vi "VISJS Viewer.vi"(4 "Extra Scripts":string, 5 "FileDependency out":map{path, T1}(c390), 6 "Options":string, 7 "OpenWebBrowser(False)":bool, 8 "error in":errorcluster, 9 "Embedd VISJS Librarya in HTMl File(False)":bool, 10 "HTMLFilePath":path, 11 "LibraryDependency":map{path, T3}(c390)) -> (0 "error out":errorcluster, 3 "HTMLFileContent":string)   [LabVIEW 2020, in "VISJS Viewer.lvlib"] (continued)
this.physicsBody,g),this.gravitySolver=new WR(this.body,this.physicsBody,g)):\"hierarchicalRepulsion\"===this.options.solver?(g=this.options.hierarchicalRepulsion,this.nodesSolver=new LR(this.body,this.physicsBody,g),this.edgesSolver=new YR(this.body,this.physicsBody,g),this.gravitySolver=new WR(this.body,this.physicsBody,g)):(g=this.options.barnesHut,this.nodesSolver=new GR(this.body,this.physicsBody,g),this.edgesSolver=new VR(this.body,this.physicsBody,g),this.gravitySolver=new WR(this.body,this.physicsBody,g)),this.modelOptions=g}},{key:\"initPhysics\",value:function(){!0===this.physicsEnabled&&!0===this.options.enabled?!0===this.options.stabilization.enabled?this.stabilize():(this.stabilized=!1,this.ready=!0,this.body.emitter.emit(\"fit\",{},this.layoutFailed),this.startSimulation()):(this.ready=!0,this.body.emitter.emit(\"fit\"))}},{key:\"startSimulation\",value:function(){var g;!0===this.physicsEnabled&&!0===this.options.enabled?(this.stabilized=!1,this.adaptiveTimestep=!1,this.body.emitter.emit(\"_resizeNodes\"),void 0===this.viewFunction&&(this.viewFunction=je(g=this.simulationStep).call(g,this),this.body.emitter.on(\"initRedraw\",this.viewFunction),this.body.emitter.emit(\"_startRendering\"))):this.body.emitter.emit(\"_redraw\")}},{key:\"stopSimulation\",value:function(){var g=!(arguments.length>0&&void 0!==arguments[0])||arguments[0];this.stabilized=!0,!0===g&&this._emitStabilized(),void 0!==this.viewFunction&&(this.body.emitter.off(\"initRedraw\",this.viewFunction),this.viewFunction=void 0,!0===g&&this.body.emitter.emit(\"_stopRendering\"))}},{key:\"simulationStep\",value:function(){var g=Qh();this.physicsTick(),(Qh()-g<.4*this.simulationInterval||!0===this.runDoubleSpeed)&&!1===this.stabilized&&(this.physicsTick(),this.runDoubleSpeed=!0),!0===this.stabilized&&this.stopSimulation()}},{key:\"_emitStabilized\",value:function(){var g=this,t=arguments.length>0&&void 0!==arguments[0]?arguments[0]:this.stabilizationIterations;(this.stabilizationIterations>1||!0===this.startedStabilization)&&wu((function(){g.body.emitter.emit(\"stabilized\",{iterations:t}),g.startedStabilization=!1,g.stabilizationIterations=0}),0)}},{key:\"physicsStep\",value:function(){this.gravitySolver.solve(),this.nodesSolver.solve(),this.edgesSolver.solve(),this.moveNodes()}},{key:\"adjustTimeStep\",value:function(){!0===this._evaluateStepQuality()?this.timestep=1.2*this.timestep:this.timestep/1.2<this.options.timestep?this.timestep=this.options.timestep:(this.adaptiveCounter=-1,this.timestep=Math.max(this.options.timestep,this.timestep/1.2))}},{key:\"physicsTick\",value:function(){if(this._startStabilizing(),!0!==this.stabilized){if(!0===this.adaptiveTimestep&&!0===this.adaptiveTimestepEnabled)this.adaptiveCounter%this.adaptiveInterval==0?(this.timestep=2*this.timestep,this.physicsStep(),this.revert(),this.timestep=.5*this.timestep,this.physicsStep(),this.physicsStep(),this.adjustTimeStep()):this.physicsStep(),this.adaptiveCounter+=1;else this.timestep=this.options.timestep,this.physicsStep();!0===this.stabilized&&this.revert(),this.stabilizationIterations++}}},{key:\"updatePhysicsData\",value:function(){this.physicsBody.forces={},this.physicsBody.physicsNodeIndices=[],this.physicsBody.physicsEdgeIndices=[];var g=this.body.nodes,t=this.body.edges;for(var A in g)Object.prototype.hasOwnProperty.call(g,A)&&!0===g[A].options.physics&&this.physicsBody.physicsNodeIndices.push(g[A].id);for(var e in t)Object.prototype.hasOwnProperty.call(t,e)&&!0===t[e].options.physics&&this.physicsBody.physicsEdgeIndices.push(t[e].id);for(var C=0;C<this.physicsBody.physicsNodeIndices.length;C++){var I=this.physicsBody.physicsNodeIndices[C];this.physicsBody.forces[I]={x:0,y:0},void 0===this.physicsBody.velocities[I]&&(this.physicsBody.velocities[I]={x:0,y:0})}for(var i in this.physicsBody.velocities)void 0===g[i]&&delete this.physicsBody.velocities[i]}},{key:\"revert\",value:function(){var g=Lh(this.previousStates),t=this.body.nodes,A=this.physicsBody.velocities;this.referenceState={};for(var e=0;e<g.length;e++){var C=g[e];void 0!==t[C]?!0===t[C].options.physics&&(this.referenceState[C]={positions:{x:t[C].x,y:t[C].y}},A[C].x=this.previousStates[C].vx,A[C].y=this.previousStates[C].vy,t[C].x=this.previousStates[C].x,t[C].y=this.previousStates[C].y):delete this.previousStates[C]}}},{key:\"_evaluateStepQuality\",value:function(){var g,t,A=this.body.nodes,e=this.referenceState;for(var C in this.referenceState)if(Object.prototype.hasOwnProperty.call(this.referenceState,C)&&void 0!==A[C]&&(g=A[C].x-e[C].positions.x,t=A[C].y-e[C].positions.y,Math.sqrt(Math.pow(g,2)+Math.pow(t,2))>.3))return!1;return!0}},{key:\"moveNodes\",value:function(){for(var g=this.physicsBody.physicsNodeIndices,t=0,A=0,e=0;e<g.length;e++){var C=g[e],I=this._performStep(C);t=Math.max(t,I),A+=I}this.adaptiveTimestepEnabled=A/g.length<5,this.stabilized=t<this.options.minVelocity}},{key:\"calculateComponentVelocity\",value:function(g,t,A){g+=(t-this.modelOptions.damping*g)/A*this.timestep;var e=this.options.maxVelocity||1e9;return Math.abs(g)>e&&(g=g>0?e:-e),g}},{key:\"_performStep\",value:function(g){var t=this.body.nodes[g],A=this.physicsBody.forces[g];this.options.wind&&(A.x+=this.options.wind.x,A.y+=this.options.wind.y);var e=this.physicsBody.velocities[g];return this.previousStates[g]={x:t.x,y:t.y,vx:e.x,vy:e.y},!1===t.options.fixed.x?(e.x=this.calculateComponentVelocity(e.x,A.x,t.options.mass),t.x+=e.x*this.timestep):(A.x=0,e.x=0),!1===t.options.fixed.y?(e.y=this.calculateComponentVelocity(e.y,A.y,t.options.mass),t.y+=e.y*this.timestep):(A.y=0,e.y=0),Math.sqrt(Math.pow(e.x,2)+Math.pow(e.y,2))}},{key:\"_freezeNodes\",value:function(){var g=this.body.nodes;for(var t in g)if(Object.prototype.hasOwnProperty.call(g,t)&&g[t].x&&g[t].y){var A=g[t].options.fixed;this.freezeCache[t]={x:A.x,y:A.y},A.x=!0,A.y=!0}}},{key:\"_restoreFrozenNodes\",value:function(){var g=this.body.nodes;for(var t in g)Object.prototype.hasOwnProperty.call(g,t)&&void 0!==this.freezeCache[t]&&(g[t].options.fixed.x=this.freezeCache[t].x,g[t].options.fixed.y=this.freezeCache[t].y);this.freezeCache={}}},{key:\"stabilize\",value:function(){var g=this,t=arguments.length>0&&void 0!==arguments[0]?arguments[0]:this.options.stabilization.iterations;\"number\"!=typeof t&&(t=this.options.stabilization.iterations,console.error(\"The stabilize method needs a numeric amount of iterations. Switching to default: \",t)),0!==this.physicsBody.physicsNodeIndices.length?(this.adaptiveTimestep=this.options.adaptiveTimestep,this.body.emitter.emit(\"_resizeNodes\"),this.stopSimulation(),this.stabilized=!1,this.body.emitter.emit(\"_blockRedraw\"),this.targetIterations=t,!0===this.options.stabilization.onlyDynamicEdges&&this._freezeNodes(),this.stabilizationIterations=0,wu((function(){return g._stabilizationBatch()}),0)):this.ready=!0}},{key:\"_startStabilizing\",value:function(){return!0!==this.startedStabilization&&(this.body.emitter.emit(\"startStabilizing\"),this.startedStabilization=!0,!0)}},{key:\"_stabilizationBatch\",value:function(){var g=this,t=function(){return!1===g.stabilized&&g.stabilizationIterations<g.targetIterations},A=function(){g.body.emitter.emit(\"stabilizationProgress\",{iterations:g.stabilizationIterations,total:g.targetIterations})};this._startStabilizing()&&A();for(var e,C=0;t()&&C<this.options.stabilization.updateInterval;)this.physicsTick(),C++;(A(),t())?wu(je(e=this._stabilizationBatch).call(e,this),0):this._finalizeStabilization()}},{key:\"_finalizeStabilization\",value:function(){this.body.emitter.emit(\"_allowRedraw\"),!0===this.options.stabilization.fit&&this.body.emitter.emit(\"fit\"),!0===this.options.stabilization.onlyDynamicEdges&&this._restoreFrozenNodes(),this.body.emitter.emit(\"stabilizationIterationsDone\"),this.body.emitter.emit(\"_requestRedraw\"),!0===this.stabilized?this._emitStabilized():this.startSimulation(),this.ready=!0}},{key:\"_drawForces\",value:function(g){for(var t=0;t<this.physicsBody.physicsNodeIndices.length;t++){var A=this.physicsBody.physicsNodeIndices[t],e=this.body.nodes[A],C=this.physicsBody.forces[A],I=Math.sqrt(Math.pow(C.x,2)+Math.pow(C.x,2)),i=Math.min(Math.max(5,I),15),o=3*i,n=nv((180-180*Math.min(1,Math.max(0,.03*I)))/360,1,1),r={x:e.x+20*C.x,y:e.y+20*C.y};g.lineWidth=i,g.strokeStyle=n,g.beginPath(),g.moveTo(e.x,e.y),g.lineTo(r.x,r.y),g.stroke();var s=Math.atan2(C.y,C.x);g.fillStyle=n,vR.draw(g,{type:\"arrow\",point:r,angle:s,length:o}),Bu(g).call(g)}}}]),g}(),XR=function(){function g(){cn(this,g)}return kd(g,null,[{key:\"getRange\",value:function(g){var t,A=arguments.length>1&&void 0!==arguments[1]?arguments[1]:[],e=1e9,C=-1e9,I=1e9,i=-1e9;if(A.length>0)for(var o=0;o<A.length;o++)I>(t=g[A[o]]).shape.boundingBox.left&&(I=t.shape.boundingBox.left),i<t.shape.boundingBox.right&&(i=t.shape.boundingBox.right),e>t.shape.boundingBox.top&&(e=t.shape.boundingBox.top),C<t.shape.boundingBox.bottom&&(C=t.shape.boundingBox.bottom);return 1e9===I&&-1e9===i&&1e9===e&&-1e9===C&&(e=0,C=0,I=0,i=0),{minX:I,maxX:i,minY:e,maxY:C}}},{key:\"getRangeCore\",value:function(g){var t,A=arguments.length>1&&void 0!==arguments[1]?arguments[1]:[],e=1e9,C=-1e9,I=1e9,i=-1e9;if(A.length>0)for(var o=0;o<A.length;o++)I>(t=g[A[o]]).x&&(I=t.x),i<t.x&&(i=t.x),e>t.y&&(e=t.y),C<t.y&&(C=t.y);return 1e9===I&&-1e9===i&&1e9===e&&-1e9===C&&(e=0,C=0,I=0,i=0),{minX:I,maxX:i,minY:e,maxY:C}}},{key:\"findCenter\",value:function(g){return{x:.5*(g.maxX+g.minX),y:.5*(g.maxY+g.minY)}}},{key:\"cloneOptions\",value:function(g,t){var A={};return void 0===t||\"node\"===t?(qf(A,g.options,!0),A.x=g.x,A.y=g.y,A.amountOfConnections=g.edges.length):qf(A,g.options,!0),A}}]),g}();function JR(g){var t=function(){if(\"undefined\"==typeof Reflect||!MT)return!1;if(MT.sham)return!1;if(\"function\"==typeof Proxy)return!0;try{return Boolean.prototype.valueOf.call(MT(Boolean,[],(function(){}))),!0}catch(g){return!1}}();return function(){var A,e=nb(g);if(t){var C=nb(this).constructor;A=MT(e,arguments,C)}else A=e.apply(this,arguments);return Ib(this,A)}}var qR=function(g){Cb(A,g);var t=JR(A);function A(g,e,C,I,i,o){var n;return cn(this,A),(n=t.call(this,g,e,C,I,i,o)).isCluster=!0,n.containedNodes={},n.containedEdges={},n}return kd(A,[{key:\"_openChildCluster\",value:function(g){var t=this,A=this.body.nodes[g];if(void 0===this.containedNodes[g])throw new Error(\"node with id: \"+g+\" not in current cluster\");if(!A.isCluster)throw new Error(\"node with id: \"+g+\" is not a cluster\");delete this.containedNodes[g],tv(A.edges,(function(g){delete t.containedEdges[g.id]})),tv(A.containedNodes,(function(g,A){t.containedNodes[A]=g})),A.containedNodes={},tv(A.containedEdges,(function(g,A){t.containedEdges[A]=g})),A.containedEdges={},tv(A.edges,(function(g){tv(t.edges,(function(A){var e,C,I=Xc(e=A.clusteringEdgeReplacingIds).call(e,g.id);-1!==I&&(tv(g.clusteringEdgeReplacingIds,(function(g){A.clusteringEdgeReplacingIds.push(g),t.body.edges[g].edgeReplacedById=A.id})),Zl(C=A.clusteringEdgeReplacingIds).call(C,I,1))}))})),A.edges=[]}}]),A}(jN),$R=function(){function g(t){var A=this;cn(this,g),this.body=t,this.clusteredNodes={},this.clusteredEdges={},this.options={},this.defaultOptions={},fe(this.options,this.defaultOptions),this.body.emitter.on(\"_resetData\",(function(){A.clusteredNodes={},A.clusteredEdges={}}))}return kd(g,[{key:\"clusterByHubsize\",value:function(g,t){void 0===g?g=this._getHubSize():\"object\"===yd(g)&&(t=this._checkOptions(g),g=this._getHubSize());for(var A=[],e=0;e<this.body.nodeIndices.length;e++){var C=this.body.nodes[this.body.nodeIndices[e]];C.edges.length>=g&&A.push(C.id)}for(var I=0;I<A.length;I++)this.clusterByConnection(A[I],t,!0);this.body.emitter.emit(\"_dataChanged\")}},{key:\"cluster\",value:function(){var g=this,t=arguments.length>0&&void 0!==arguments[0]?arguments[0]:{},A=!(arguments.length>1&&void 0!==arguments[1])||arguments[1];if(void 0===t.joinCondition)throw new Error(\"Cannot call clusterByNodeData without a joinCondition function in the options.\");t=this._checkOptions(t);var e={},C={};tv(this.body.nodes,(function(A,I){A.options&&!0===t.joinCondition(A.options)&&(e[I]=A,tv(A.edges,(function(t){void 0===g.clusteredEdges[t.id]&&(C[t.id]=t)})))})),this._cluster(e,C,t,A)}},{key:\"clusterByEdgeCount\",value:function(g,t){var A=this,e=!(arguments.length>2&&void 0!==arguments[2])||arguments[2];t=this._checkOptions(t);for(var C,I,i,o=[],n={},r=function(){var e={},r={},a=A.body.nodeIndices[s],d=A.body.nodes[a];if(void 0===n[a]){i=0,I=[];for(var h=0;h<d.edges.length;h++)C=d.edges[h],void 0===A.clusteredEdges[C.id]&&(C.toId!==C.fromId&&i++,I.push(C));if(i===g){for(var l=function(g){if(void 0===t.joinCondition||null===t.joinCondition)return!0;var A=XR.cloneOptions(g);return t.joinCondition(A)},c=!0,u=0;u<I.length;u++){C=I[u];var p=A._getConnectedId(C,a);if(!l(d)){c=!1;break}r[C.id]=C,e[a]=d,e[p]=A.body.nodes[p],n[a]=!0}if(Lh(e).length>0&&Lh(r).length>0&&!0===c){var f=function(){for(var g=0;g<o.length;++g)for(var t in e)if(void 0!==o[g].nodes[t])return o[g]}();if(void 0!==f){for(var v in e)void 0===f.nodes[v]&&(f.nodes[v]=e[v]);for(var y in r)void 0===f.edges[y]&&(f.edges[y]=r[y])}else o.push({nodes:e,edges:r})}}}},s=0;s<this.body.nodeIndices.length;s++)r();for(var a=0;a<o.length;a++)this._cluster(o[a].nodes,o[a].edges,t,!1);!0===e&&this.body.emitter.emit(\"_dataChanged\")}},{key:\"clusterOutliers\",value:function(g){var t=!(arguments.length>1&&void 0!==arguments[1])||arguments[1];this.clusterByEdgeCount(1,g,t)}},{key:\"clusterBridges\",value:function(g){var t=!(arguments.length>1&&void 0!==arguments[1])||arguments[1];this.clusterByEdgeCount(2,g,t)}},{key:\"clusterByConnection\",value:function(g,t){var A,e=!(arguments.length>2&&void 0!==arguments[2])||arguments[2];if(void 0===g)throw new Error(\"No nodeId supplied to clusterByConnection!\");if(void 0===this.body.nodes[g])throw new Error(\"The nodeId given to clusterByConnection does not exist!\");var C=this.body.nodes[g];void 0===(t=this._checkOptions(t,C)).clusterNodeProperties.x&&(t.clusterNodeProperties.x=C.x),void 0===t.clusterNodeProperties.y&&(t.clusterNodeProperties.y=C.y),void 0===t.clusterNodeProperties.fixed&&(t.clusterNodeProperties.fixed={},t.clusterNodeProperties.fixed.x=C.options.fixed.x,t.clusterNodeProperties.fixed.y=C.options.fixed.y);var I={},i={},o=C.id,n=XR.cloneOptions(C);I[o]=C;for(var r=0;r<C.edges.length;r++){var s=C.edges[r];if(void 0===this.clusteredEdges[s.id]){var a=this._getConnectedId(s,o);if(void 0===this.clusteredNodes[a])if(a!==o)if(void 0===t.joinCondition)i[s.id]=s,I[a]=this.body.nodes[a];else{var d=XR.cloneOptions(this.body.nodes[a]);!0===t.joinCondition(n,d)&&(i[s.id]=s,I[a]=this.body.nodes[a])}else i[s.id]=s}}var h=Fh(A=Lh(I)).call(A,(function(g){return I[g].id}));for(var l in I)if(Object.prototype.hasOwnProperty.call(I,l))for(var c=I[l],u=0;u<c.edges.length;u++){var p=c.edges[u];Xc(h).call(h,this._getConnectedId(p,c.id))>-1&&(i[p.id]=p)}this._cluster(I,i,t,e)}},{key:\"_createClusterEdges\",value:function(g,t,A,e){for(var C,I,i,o,n,r,s=Lh(g),a=[],d=0;d<s.length;d++){i=g[I=s[d]];for(var h=0;h<i.edges.length;h++)C=i.edges[h],void 0===this.clusteredEdges[C.id]&&(C.toId==C.fromId?t[C.id]=C:C.toId==I?(o=A.id,r=n=C.fromId):(o=C.toId,n=A.id,r=o),void 0===g[r]&&a.push({edge:C,fromId:n,toId:o}))}for(var l=[],c=function(g){for(var t=0;t<l.length;t++){var A=l[t],e=g.fromId===A.fromId&&g.toId===A.toId,C=g.fromId===A.toId&&g.toId===A.fromId;if(e||C)return A}return null},u=0;u<a.length;u++){var p=a[u],f=p.edge,v=c(p);null===v?(v=this._createClusteredEdge(p.fromId,p.toId,f,e),l.push(v)):v.clusteringEdgeReplacingIds.push(f.id),this.body.edges[f.id].edgeReplacedById=v.id,this._backupEdgeOptions(f),f.setOptions({physics:!1})}}},{key:\"_checkOptions\",value:function(){var g=arguments.length>0&&void 0!==arguments[0]?arguments[0]:{};return void 0===g.clusterEdgeProperties&&(g.clusterEdgeProperties={}),void 0===g.clusterNodeProperties&&(g.clusterNodeProperties={}),g}},{key:\"_cluster\",value:function(g,t,A){var e=!(arguments.length>3&&void 0!==arguments[3])||arguments[3],C=[];for(var I in g)Object.prototype.hasOwnProperty.call(g,I)&&void 0!==this.clusteredNodes[I]&&C.push(I);for(var i=0;i<C.length;++i)delete g[C[i]];if(0!=Lh(g).length&&(1!=Lh(g).length||1==A.clusterNodeProperties.allowSingleNodeCluster)){var o=qf({},A.clusterNodeProperties);if(void 0!==A.processProperties){var n=[];for(var r in g)if(Object.prototype.hasOwnProperty.call(g,r)){var s=XR.cloneOptions(g[r]);n.push(s)}var a=[];for(var d in t)if(Object.prototype.hasOwnProperty.call(t,d)&&\"clusterEdge:\"!==d.substr(0,12)){var h=XR.cloneOptions(t[d],\"edge\");a.push(h)}if(!(o=A.processProperties(o,n,a)))throw new Error(\"The processProperties function does not return properties!\")}void 0===o.id&&(o.id=\"cluster:\"+rD());var l=o.id;void 0===o.label&&(o.label=\"cluster\");var c=void 0;void 0===o.x&&(c=this._getClusterPosition(g),o.x=c.x),void 0===o.y&&(void 0===c&&(c=this._getClusterPosition(g)),o.y=c.y),o.id=l;var u=this.body.functions.createNode(o,qR);u.containedNodes=g,u.containedEdges=t,u.clusterEdgeProperties=A.clusterEdgeProperties,this.body.nodes[o.id]=u,this._clusterEdges(g,t,o,A.clusterEdgeProperties),o.id=void 0,!0===e&&this.body.emitter.emit(\"_dataChanged\")}}},{key:\"_backupEdgeOptions\",value:function(g){void 0===this.clusteredEdges[g.id]&&(this.clusteredEdges[g.id]={physics:g.options.physics})}},{key:\"_restoreEdge\",value:function(g){var t=this.clusteredEdges[g.id];void 0!==t&&(g.setOptions({physics:t.physics}),delete this.clusteredEdges[g.id])}},{key:\"isCluster\",value:function(g){return void 0!==this.body.nodes[g]?!0===this.body.nodes[g].isCluster:(console.error(\"Node does not exist.\"),!1)}},{key:\"_getClusterPosition\",value:function(g){for(var t,A=Lh(g),e=g[A[0]].x,C=g[A[0]].x,I=g[A[0]].y,i=g[A[0]].y,o=1;o<A.length;o++)e=(t=g[A[o]]).x<e?t.x:e,C=t.x>C?t.x:C,I=t.y<I?t.y:I,i=t.y>i?t.y:i;return{x:.5*(e+C),y:.5*(I+i)}}},{key:\"openCluster\",value:function(g,t){var A=!(arguments.length>2&&void 0!==arguments[2])||arguments[2];if(void 0===g)throw new Error(\"No clusterNodeId supplied to openCluster.\");var e=this.body.nodes[g];if(void 0===e)throw new Error(\"The clusterNodeId supplied to openCluster does not exist.\");if(!0!==e.isCluster||void 0===e.containedNodes||void 0===e.containedEdges)throw new Error(\"The node:\"+g+\" is not a valid cluster.\");var C=this.findNode(g),I=Xc(C).call(C,g)-1;if(I>=0){var i=C[I];return this.body.nodes[i]._openChildCluster(g),delete this.body.nodes[g],void(!0===A&&this.body.emitter.emit(\"_dataChanged\"))}var o=e.containedNodes,n=e.containedEdges;if(void 0!==t&&void 0!==t.releaseFunction&&\"function\"==typeof t.releaseFunction){var r={},s={x:e.x,y:e.y};for(var a in o)if(Object.prototype.hasOwnProperty.call(o,a)){var d=this.body.nodes[a];r[a]={x:d.x,y:d.y}}var h=t.releaseFunction(s,r);for(var l in o)if(Object.prototype.hasOwnProperty.call(o,l)){var c=this.body.nodes[l];void 0!==h[l]&&(c.x=void 0===h[l].x?e.x:h[l].x,c.y=void 0===h[l].y?e.y:h[l].y)}}else tv(o,(function(g){!1===g.options.fixed.x&&(g.x=e.x),!1===g.options.fixed.y&&(g.y=e.y)}));for(var u in o)if(Object.prototype.hasOwnProperty.call(o,u)){var p=this.body.nodes[u];p.vx=e.vx,p.vy=e.vy,p.setOptions({physics:!0}),delete this.clusteredNodes[u]}for(var f=[],v=0;v<e.edges.length;v++)f.push(e.edges[v]);for(var y=0;y<f.length;y++){for(var m=f[y],b=this._getConnectedId(m,g),w=this.clusteredNodes[b],k=0;k<m.clusteringEdgeReplacingIds.length;k++){var x=m.clusteringEdgeReplacingIds[k],E=this.body.edges[x];if(void 0!==E)if(void 0!==w){var O=this.body.nodes[w.clusterId];O.containedEdges[E.id]=E,delete n[E.id];var T=E.fromId,D=E.toId;E.toId==b?D=w.clusterId:T=w.clusterId,this._createClusteredEdge(T,D,E,O.clusterEdgeProperties,{hidden:!1,physics:!0})}else this._restoreEdge(E)}m.remove()}for(var N in n)Object.prototype.hasOwnProperty.call(n,N)&&this._restoreEdge(n[N]);delete this.body.nodes[g],!0===A&&this.body.emitter.emit(\"_dataChanged\")}},{key:\"getNodesInCluster\",value:function(g){var t=[];if(!0===this.isCluster(g)){var 
